vi "ELVIS III v1.0 Configure Encoder.vi"(8 "error in (no error)":errorcluster, 9 "Encoder Configuration v1.0":T1, 10 "Encoder Channel":T5, 11 "myRIO Ref In":T3) -> (0 "error out":errorcluster)   [LabVIEW 2021]
uses:
  <vilib>/myRIO/Common/Instrument Driver Framework/myRIO v1.0/Encoder/typedefs/Encoder Channels Enum.ctl
  <vilib>/myRIO/Common/Instrument Driver Framework/Utilities/typedefs/myRIO v1.0 Reference.ctl
  <vilib>/myRIO/Common/Instrument Driver Framework/Utilities/typedefs/Generic FPGA Reference.ctl
  <vilib>/myRIO/Common/Instrument Driver Framework/myRIO v1.0/Encoder/typedefs/Encoder Configuration v1.0.ctl
  <vilib>/myRIO/Common/Instrument Driver Framework/myRIO v1.0/Encoder/typedefs/Encoder Signal Mode.ctl
  <vilib>/myRIO/Common/Instrument Driver Framework/myRIO v1.0/Encoder/typedefs/Encoder Config Manager Action Enum.ctl
  <vilib>/myRIO/Common/Instrument Driver Framework/ELVIS III v1.0/Encoder/typedefs/ELVIS III Encoder Channels FPGA Reference.ctl
  <vilib>/rvi/errors/niLvFpgaAdjustHostInterfaceError.vi
  <vilib>/rvi/interface/nirviReadWriteControl/nirviReadWriteControl.xnode
  NiFpgaLv.dll
  <vilib>/rvi/interface/Simulation/niFpgaSimulationCallBeginRW.vi
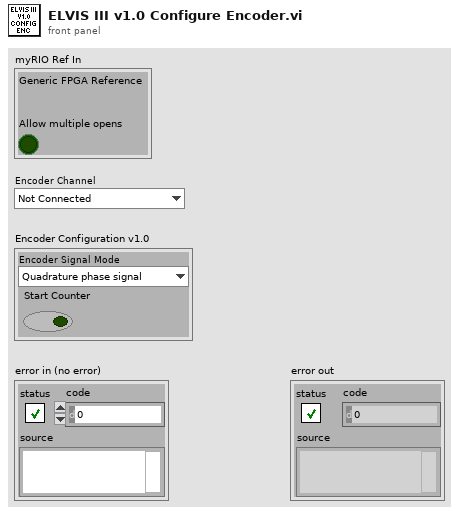
[diagram p1: front panel]
types:
  T1 = typedef "Encoder Configuration v1.0.ctl" = cluster{"Encoder Signal Mode":T2, "Start Counter":bool}
  T2 = typedef "Encoder Signal Mode.ctl" = enum16{"Quadrature phase signal", "Step and direction signal"}
  T3 = typedef "myRIO v1.0 Reference.ctl" = cluster{"Generic FPGA Reference":T4, "Allow multiple opens":bool}
  T4 = typedef "Generic FPGA Reference.ctl" = refnum<k20>
  T5 = typedef "Encoder Channels Enum.ctl" = enum16{"Not Connected", "C/ENC0", "C/ENC1", "A/ENC", "A/ENC0", "A/ENC1", "A/ENC2", "A/ENC3", "A/ENC4", "A/ENC5", "A/ENC6", "A/ENC7", "A/ENC8", "A/ENC9", "B/ENC", "B/ENC0", "B/ENC1", "B/ENC2", "B/ENC3", "B/ENC4", "B/ENC5", "B/ENC6", "B/ENC7", "B/ENC8", "B/ENC9", "DIO/ENC0", "DIO/ENC1", "DIO/ENC2", "DIO/ENC3", "DIO/ENC4"}
  T6 = typedef "Encoder Config Manager Action Enum.ctl" = enum16{"Do Nothing", "Store", "Clear"}
  T7 = typedef "ELVIS III Encoder Channels FPGA Reference.ctl" = refnum<k20>
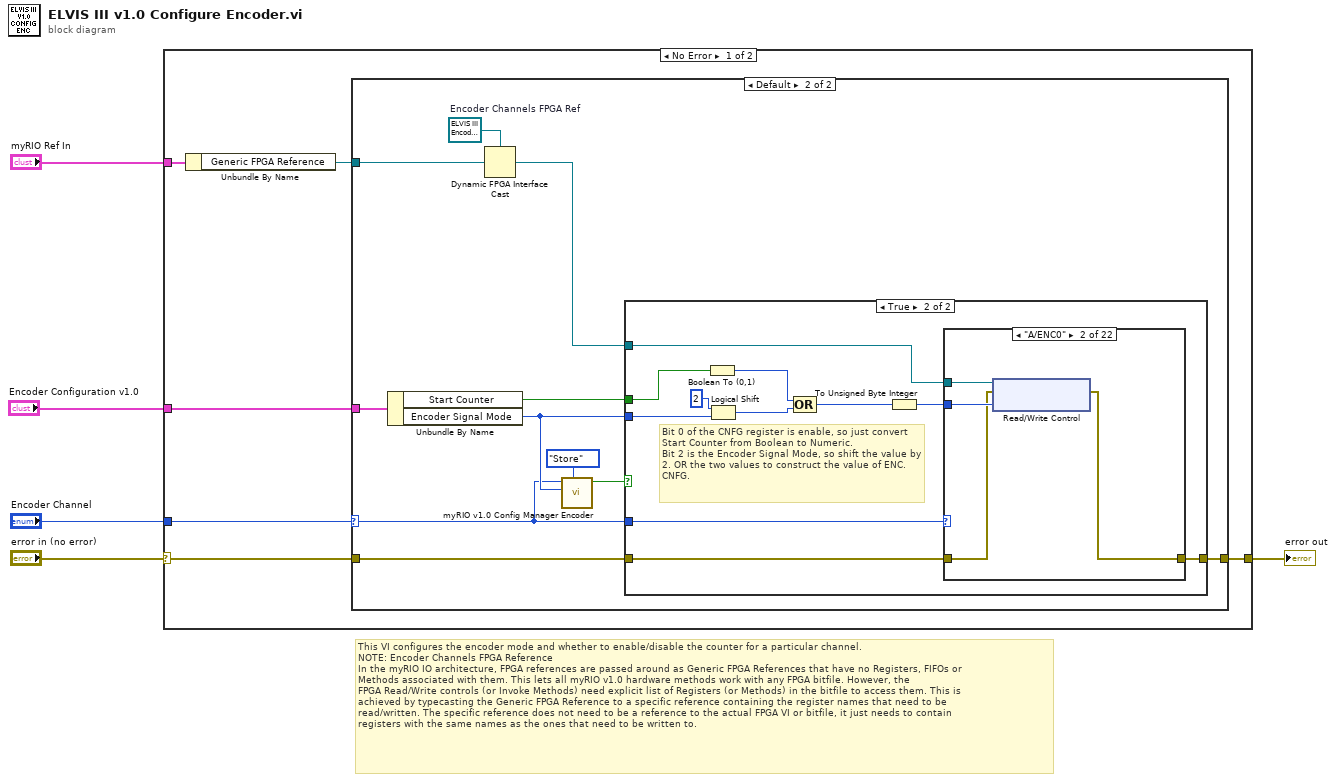
[diagram p0: block diagram]
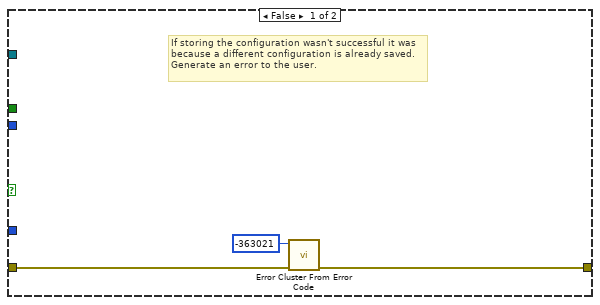
[diagram p3: hidden frame]
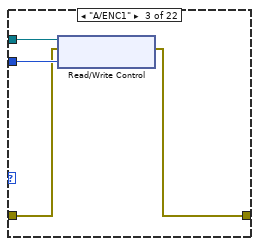
[diagram p5: hidden frame]
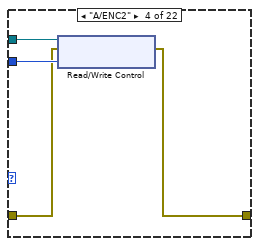
[diagram p6: hidden frame]
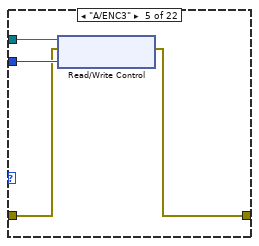
[diagram p7: hidden frame]
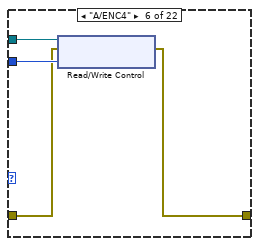
[diagram p8: hidden frame]
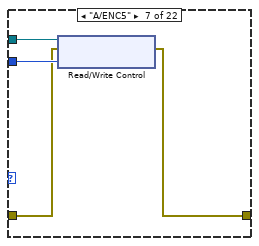
[diagram p9: hidden frame]
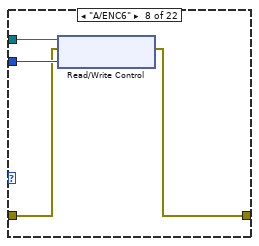
[diagram p10: hidden frame]
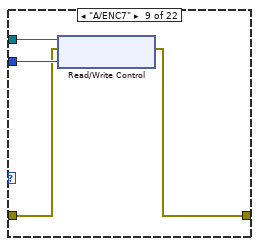
[diagram p11: hidden frame]
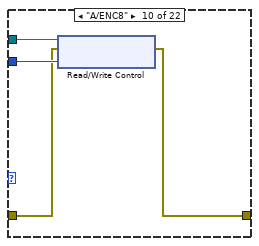
[diagram p12: hidden frame]
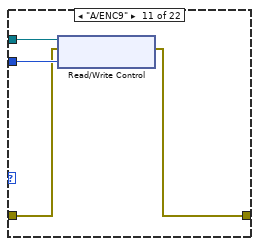
[diagram p13: hidden frame]
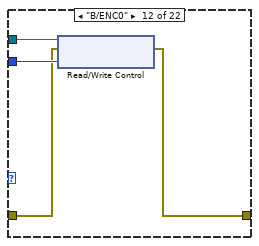
[diagram p14: hidden frame]
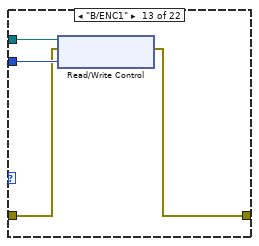
[diagram p15: hidden frame]
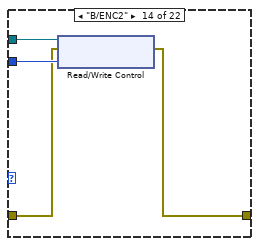
[diagram p16: hidden frame]
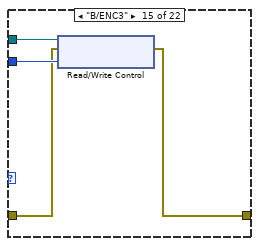
[diagram p17: hidden frame]
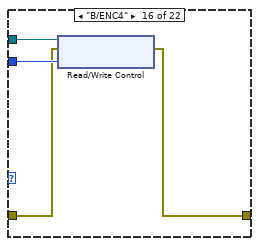
[diagram p18: hidden frame]
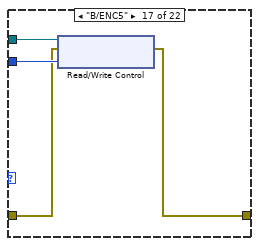
[diagram p19: hidden frame]
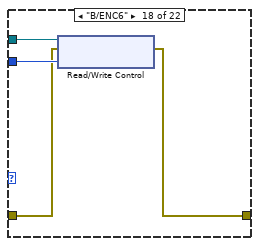
[diagram p20: hidden frame]
diagram:
  # "This VI configures the encoder mode and whether to enable/disable the counter for a particular channel.\nNOTE: Encoder Channels FPGA Reference\nIn the myRIO IO architecture, FPGA references are passed around as Generic FPGA References that have no Registers, FIFOs or\nMethods associated with them. This lets all myRIO v1.0 hardware methods work with any FPGA bitfile. However, the \nFPGA Read/Write controls (or Invoke Methods) need explicit list of Registers (or Methods) in the bitfile to access them. This is \nachieved by typecasting the Generic FPGA Reference to a specific reference containing the register names that need to be \nread/written. The specific reference does not need to be a reference to the actual FPGA VI or bitfile, it just needs to contain \nregisters with the same names as the ones that need to be written to."
  n1 = case shown="No Error" "error in (no error)" {
    selector: "error in (no error)" -> [w10 w122]
    tunnel: [w11 w122] -> w5
    tunnel: "myRIO Ref In" -> [w9 _]
    tunnel: "Encoder Channel" -> [w8 _]
    tunnel: "Encoder Configuration v1.0" -> [w7 _]
    frame No Error {
      n2 = Unbundle By Name(w9) -> ("Generic FPGA Reference"=w6:T4)
      n3 = case shown="Default" w8 {
        selector: w8 -> [_ w14]
        tunnel: [w12 w21] -> w11
        tunnel: w10 -> [w12 w20]
        tunnel: w6 -> [_ w19]
        tunnel: w7 -> [_ w18]
        frame "Not Connected" {
        }
        frame Default {
          w23 = T7 refnum  # Encoder Channels FPGA Ref
          n4 = Unbundle By Name(w18) -> ("Start Counter"=w17:bool, "Encoder Signal Mode"=w15:T2)
          n5 = Dynamic FPGA Interface Cast(Session In=w23, Type=w19) -> (Session Out=w22:T7)
          n6 = call <vilib>:"myRIO v1.0 Config Manager Encoder.vi"("Action"=Encoder_Config_Manager_Action_Enum."Store", "Encoder Signal Mode"=w15, "Encoder Channel"=w14) -> ("Success?"=w13:bool)  [unwired: 8 in]
          n7 = case shown="True" w13 {
            tunnel: w22 -> [_ w37]
            tunnel: [w25 w36] -> w21
            tunnel: w20 -> [w26 w35]
            tunnel: w17 -> [_ w32]
            tunnel: w15 -> [_ w28]
            tunnel: w14 -> [_ w27]
            frame False {
              # "If storing the configuration wasn't successful it was because a different configuration is already saved. Generate an error to the user."
              n8 = call <vilib>:"Error Cluster From Error Code.vi"("error in (no error)"=w26, "error code (0)"=-363021) -> ("error out"=w25:errorcluster)  [unwired: 7 in]
            }
            frame True {
              # "Bit 0 of the CNFG register is enable, so just convert Start Counter from Boolean to Numeric.\nBit 2 is the Encoder Signal Mode, so shift the value by 2. OR the two values to construct the value of ENC.CNFG."
              n9 = Boolean To (0,1)(Boolean=w32) -> (0, 1=w31:i16)
              n10 = Logical Shift(y=i8 2, x=w28) -> (x << y=w29:u32)
              n11 = Compound Arithmetic op=OR(w31, w29) -> (w30:u32)
              n12 = To Unsigned Byte Integer(number=w30) -> (unsigned 8bit integer=w33:u8)
              n13 = case shown="\"A/ENC0\"" w27 {
                tunnel: w35 -> [w38 w40 w44 w48 w52 w56 w60 w64 w68 w72 w76 w80 w84 w88 w92 w96 w100 w104 w108 w112 w116 w119]
                tunnel: [w38 w39 w43 w47 w51 w55 w59 w63 w67 w71 w75 w79 w83 w87 w91 w95 w99 w103 w107 w111 w115 w120] -> w36
                tunnel: w37 -> [_ w42 w46 w50 w54 w58 w62 w66 w70 w74 w78 w82 w86 w90 w94 w98 w102 w106 w110 w114 w118 _]
                tunnel: w33 -> [_ w41 w45 w49 w53 w57 w61 w65 w69 w73 w77 w81 w85 w89 w93 w97 w101 w105 w109 w113 w117 _]
                frame "Not Connected" {
                }
                frame "A/ENC0" {
                  n14 = xnode "Read/Write Control"("FPGA VI Reference In"=w42, "error in"=w40, "ENC.A_0.CNFG"=w41) -> ("error out"=w39:errorcluster)  [unwired: 1 out]
                }
                frame "A/ENC1" {
                  n15 = xnode "Read/Write Control"("FPGA VI Reference In"=w46, "error in"=w44, "ENC.A_1.CNFG"=w45) -> ("error out"=w43:errorcluster)  [unwired: 1 out]
                }
                frame "A/ENC2" {
                  n16 = xnode "Read/Write Control"("FPGA VI Reference In"=w50, "error in"=w48, "ENC.A_2.CNFG"=w49) -> ("error out"=w47:errorcluster)  [unwired: 1 out]
                }
                frame "A/ENC3" {
                  n17 = xnode "Read/Write Control"("FPGA VI Reference In"=w54, "error in"=w52, "ENC.A_3.CNFG"=w53) -> ("error out"=w51:errorcluster)  [unwired: 1 out]
                }
                frame "A/ENC4" {
                  n18 = xnode "Read/Write Control"("FPGA VI Reference In"=w58, "error in"=w56, "ENC.A_4.CNFG"=w57) -> ("error out"=w55:errorcluster)  [unwired: 1 out]
                }
                frame "A/ENC5" {
                  n19 = xnode "Read/Write Control"("FPGA VI Reference In"=w62, "error in"=w60, "ENC.A_5.CNFG"=w61) -> ("error out"=w59:errorcluster)  [unwired: 1 out]
                }
                frame "A/ENC6" {
                  n20 = xnode "Read/Write Control"("FPGA VI Reference In"=w66, "error in"=w64, "ENC.A_6.CNFG"=w65) -> ("error out"=w63:errorcluster)  [unwired: 1 out]
                }
                frame "A/ENC7" {
                  n21 = xnode "Read/Write Control"("FPGA VI Reference In"=w70, "error in"=w68, "ENC.A_7.CNFG"=w69) -> ("error out"=w67:errorcluster)  [unwired: 1 out]
                }
                frame "A/ENC8" {
                  n22 = xnode "Read/Write Control"("FPGA VI Reference In"=w74, "error in"=w72, "ENC.A_8.CNFG"=w73) -> ("error out"=w71:errorcluster)  [unwired: 1 out]
                }
                frame "A/ENC9" {
                  n23 = xnode "Read/Write Control"("FPGA VI Reference In"=w78, "error in"=w76, "ENC.A_9.CNFG"=w77) -> ("error out"=w75:errorcluster)  [unwired: 1 out]
                }
                frame "B/ENC0" {
                  n24 = xnode "Read/Write Control"("FPGA VI Reference In"=w82, "error in"=w80, "ENC.B_0.CNFG"=w81) -> ("error out"=w79:errorcluster)  [unwired: 1 out]
                }
                frame "B/ENC1" {
                  n25 = xnode "Read/Write Control"("FPGA VI Reference In"=w86, "error in"=w84, "ENC.B_1.CNFG"=w85) -> ("error out"=w83:errorcluster)  [unwired: 1 out]
                }
                frame "B/ENC2" {
                  n26 = xnode "Read/Write Control"("FPGA VI Reference In"=w90, "error in"=w88, "ENC.B_2.CNFG"=w89) -> ("error out"=w87:errorcluster)  [unwired: 1 out]
                }
                frame "B/ENC3" {
                  n27 = xnode "Read/Write Control"("FPGA VI Reference In"=w94, "error in"=w92, "ENC.B_3.CNFG"=w93) -> ("error out"=w91:errorcluster)  [unwired: 1 out]
                }
                frame "B/ENC4" {
                  n28 = xnode "Read/Write Control"("FPGA VI Reference In"=w98, "error in"=w96, "ENC.B_4.CNFG"=w97) -> ("error out"=w95:errorcluster)  [unwired: 1 out]
                }
                frame "B/ENC5" {
                  n29 = xnode "Read/Write Control"("FPGA VI Reference In"=w102, "error in"=w100, "ENC.B_5.CNFG"=w101) -> ("error out"=w99:errorcluster)  [unwired: 1 out]
                }
                frame "B/ENC6" {
                  n30 = xnode "Read/Write Control"("FPGA VI Reference In"=w106, "error in"=w104, "ENC.B_6.CNFG"=w105) -> ("error out"=w103:errorcluster)  [unwired: 1 out]
                }
                frame "B/ENC7" {
                  n31 = xnode "Read/Write Control"("FPGA VI Reference In"=w110, "error in"=w108, "ENC.B_7.CNFG"=w109) -> ("error out"=w107:errorcluster)  [unwired: 1 out]
                }
                frame "B/ENC8" {
                  n32 = xnode "Read/Write Control"("FPGA VI Reference In"=w114, "error in"=w112, "ENC.B_8.CNFG"=w113) -> ("error out"=w111:errorcluster)  [unwired: 1 out]
                }
                frame "B/ENC9" {
                  n33 = xnode "Read/Write Control"("FPGA VI Reference In"=w118, "error in"=w116, "ENC.B_9.CNFG"=w117) -> ("error out"=w115:errorcluster)  [unwired: 1 out]
                }
                frame Default {
                  # "The channel requested is not supported. This happens when the channel name is valid (a valid channel enum) but there it is not handled in the case structure."
                  n34 = call <vilib>:"Error Cluster From Error Code.vi"("error in (no error)"=w119, "error code (0)"=-363003) -> ("error out"=w120:errorcluster)  [unwired: 7 in]
                }
              }
            }
          }
        }
      }
    }
    frame Error {
      # "There is an incoming error so there is nothing to do."
    }
  }
  "error out" <- w5
